vi "Set Data.vi"(8 "error in (no error)":errorcluster, 9 "Set Value":string, 10 "LogicName":string, 11 "PLC_Module in":refnum<class "PLC_Module.lvclass">) -> (0 "error out":errorcluster, 3 "PLC_Module out":refnum<class "PLC_Module.lvclass">)   [LabVIEW 2025, in "PLC_Module.lvlib" / "PLC_Module.lvclass"]
uses:
  PLC_Module.lvclass
  PLC_Module.lvclass/PLC_Module.ctl
  <vilib>/Utility/miscctls.llb/LVMapReplaceAction.ctl
  PLC_Abstr/PLC_Abstr Messages/Write Data Msg/Write Data Msg.lvclass/Write Data Msg.ctl
  <vilib>/ActorFramework/Message Enqueuer/Message Enqueuer.lvclass/Message Enqueuer.ctl
  b9a00cdf-f003-4314-8ef1-cc05cebe1eef.vi
  6056e4c1-ed78-404a-9ef6-920044df1d88.vi
  96e6804c-cbe1-4d7e-8e4f-31ab62afd4e7.vi
  108bd21b-5831-41ec-9599-3e5880a8ed08.vi
  effe1758-f8e4-496e-af8d-4484fbab5602.vi
  549d32eb-c80e-4b94-81c6-920abf9741ef.vi
  Write Configuration.vi
  Read Configuration.vi
  Read Connect.vi
  <vilib>/ActorFramework/Message Enqueuer/Enqueue.vi
  PLC_Abstr/PLC_Abstr Messages/Write Data Msg/Write Data Msg.lvclass
  <vilib>/JDP Science/JSONtext/JSON text to Variant.vi
  <vilib>/ActorFramework/Message Priority Queue/Priority Enqueue.vi
  <vilib>/JDP Science/JSONtext/LVClass Serializer/JSONtext LVClass Serializer.lvclass
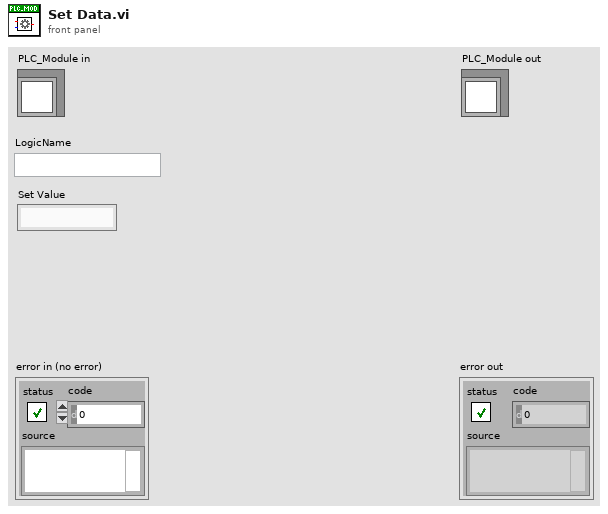
[diagram p1: front panel]
types:
  T1 = typedef "LVMapReplaceAction.ctl" = enum32{"Modify Entry only if found", "Add or Modify Entry", "Delete Entry"}
  T2 = typedef "PLC_Module.lvlib/PLC_Module.lvclass/PLC_Data_Config.ctl" = map{string, cluster{"Config":T3, "Get Value":string, "Set Value":string}}
  T3 = typedef "PLC_Module.lvlib/PLC_Module.lvclass/PLC_Data.ctl" = cluster{"Address":string, "Direction":enum16{"PC->PLC", "PLC->PC"}, "DataType":T4, "Description":string}
  T4 = typedef "PLC_Module.lvlib/PLC_Module.lvclass/PLC_Data_Type.ctl" = enum16{"Boolean", "Single Float", "U8", "U32", "U32_Array", "String"}
  T5 = cluster{"Config":T3, "Get Value":string, "Set Value":string}
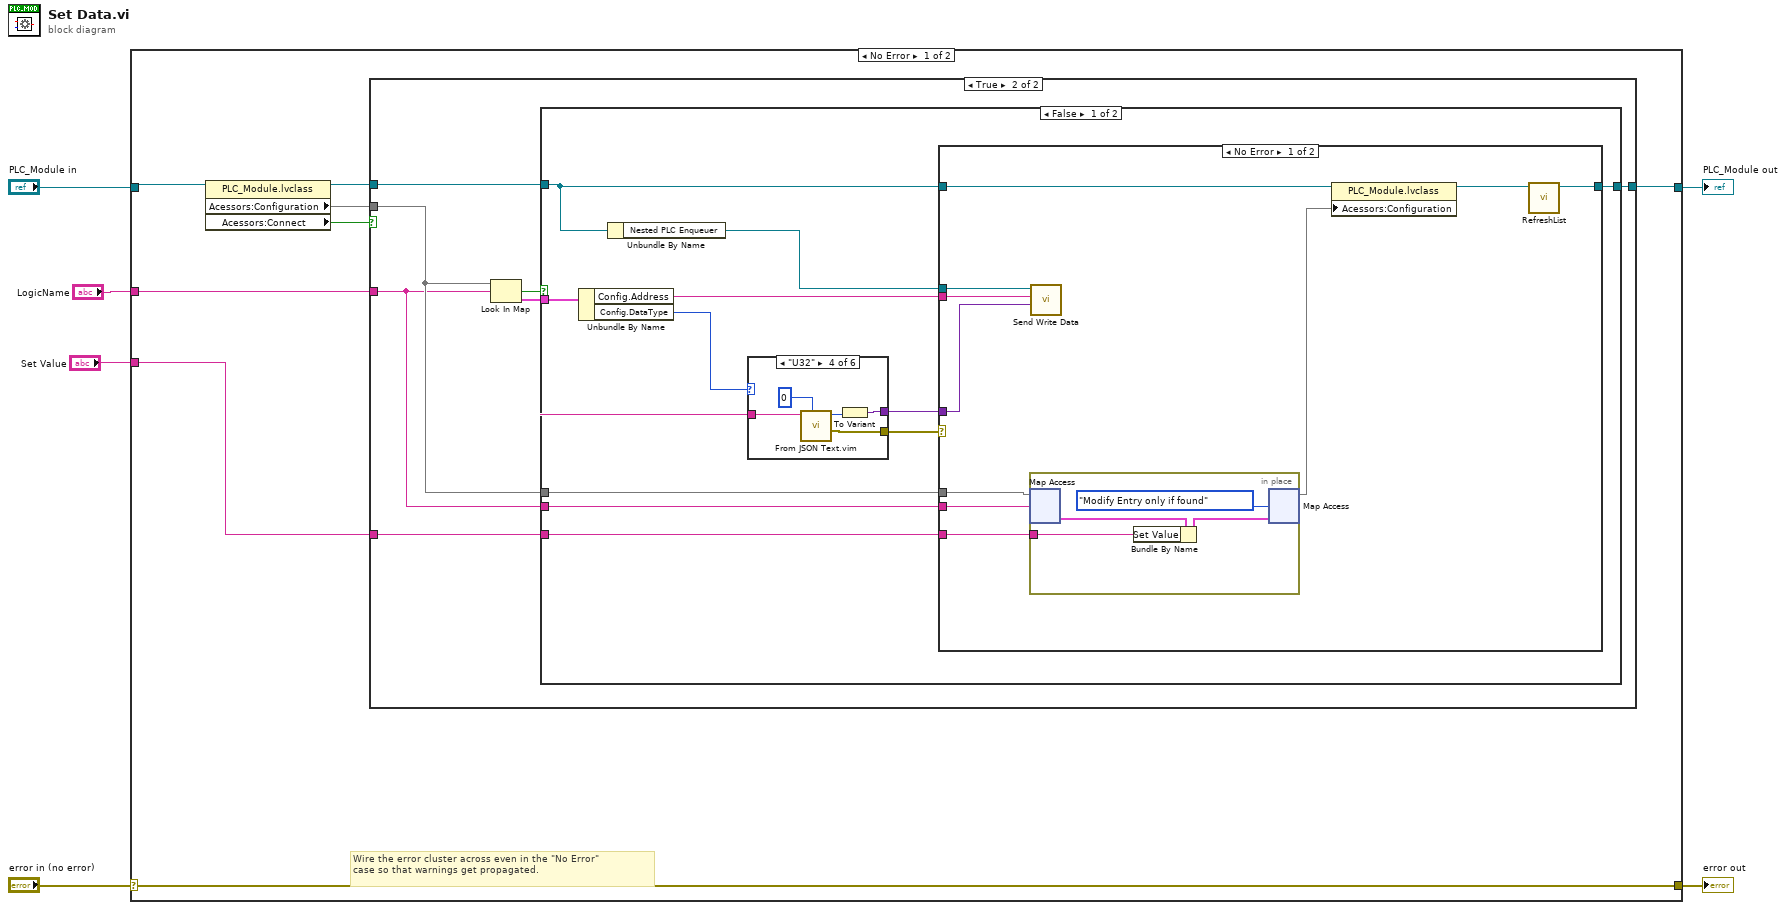
[diagram p0: block diagram]
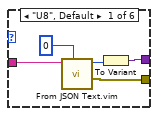
[diagram p4: hidden frame]
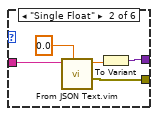
[diagram p5: hidden frame]
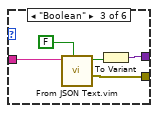
[diagram p6: hidden frame]
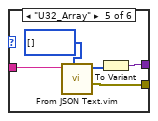
[diagram p7: hidden frame]
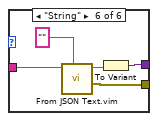
[diagram p8: hidden frame]
diagram:
  n1 = case shown="No Error" "error in (no error)" {
    selector: "error in (no error)" -> [w14 w81]
    tunnel: [w14 w81] -> w5
    tunnel: [w10 w80] -> w3
    tunnel: "PLC_Module in" -> [w13 w80]
    tunnel: "LogicName" -> [w9 _]
    tunnel: "Set Value" -> [w8 _]
    frame No Error {
      # "Wire the error cluster across even in the \"No Error\"\ncase so that warnings get propagated."
      n2 = property class="PLC_Module.lvclass"(reference=w13) -> (reference out=w12:refnum<class "PLC_Module.lvclass">, "Acessors:Configuration"=w11:T2, "Acessors:Connect"=w7:bool)  [unwired: 1 in, 1 out]
      n3 = case shown="True" w7 {
        tunnel: w12 -> [w15 w21]
        tunnel: w11 -> [_ w20]
        tunnel: [w15 w19] -> w10
        tunnel: w9 -> [_ w18]
        tunnel: w8 -> [_ w17]
        frame False {
        }
        frame True {
          n4 = Look In Map(map=w20, key=w18) -> (key not found?=w16:bool, value=w22:T5)  [unwired: 1 in]
          n5 = case shown="False" w16 {
            tunnel: w22 -> [w32 _]
            tunnel: w21 -> [w27 w79]
            tunnel: w20 -> [w26 _]
            tunnel: [w25 w79] -> w19
            tunnel: w18 -> [w24 _]
            tunnel: w17 -> [w23 _]
            frame False {
              n6 = Unbundle By Name(w32) -> ("Config.Address"=w31:string, "Config.DataType"=w30:T4)
              n7 = Unbundle By Name(w27) -> ("Nested PLC Enqueuer"=w33:refnum<class "Message Enqueuer.lvclass">)
              n8 = case shown="\"U32\"" w30 {
                tunnel: [w52 w57 w62 w67 w72 w77] -> w29
                tunnel: w23 -> [w53 w58 w63 w68 w73 w78]
                tunnel: [w49 w54 w59 w64 w70 w75] -> w28
                frame "U8", Default {
                  n9 = call "From JSON Text.vim"("Data Type and Default Value"=u8 0, "JSON"=w53) -> ("error out"=w52:errorcluster, "Data out"=w50:u8)  [unwired: 8 in]
                  n10 = To Variant(anything=w50) -> (Variant=w49:variant)
                }
                frame "Single Float" {
                  n11 = call "From JSON Text.vim"("Data Type and Default Value"=sgl 0.0, "JSON"=w58) -> ("error out"=w57:errorcluster, "Data out"=w55:sgl)  [unwired: 8 in]
                  n12 = To Variant(anything=w55) -> (Variant=w54:variant)
                }
                frame "Boolean" {
                  n13 = call "From JSON Text.vim"("Data Type and Default Value"=FALSE, "JSON"=w63) -> ("error out"=w62:errorcluster, "Data out"=w60:bool)  [unwired: 8 in]
                  n14 = To Variant(anything=w60) -> (Variant=w59:variant)
                }
                frame "U32" {
                  n15 = call "From JSON Text.vim"("Data Type and Default Value"=u32 0, "JSON"=w68) -> ("error out"=w67:errorcluster, "Data out"=w65:u32)  [unwired: 8 in]
                  n16 = To Variant(anything=w65) -> (Variant=w64:variant)
                }
                frame "U32_Array" {
                  n17 = call "From JSON Text.vim"("Data Type and Default Value"=u32[] [], "JSON"=w73) -> ("error out"=w72:errorcluster, "Data out"=w71:u32[])  [unwired: 8 in]
                  n18 = To Variant(anything=w71) -> (Variant=w70:variant)
                }
                frame "String" {
                  n19 = call "From JSON Text.vim"("Data Type and Default Value"="", "JSON"=w78) -> ("error out"=w77:errorcluster, "Data out"=w76:string)  [unwired: 8 in]
                  n20 = To Variant(anything=w76) -> (Variant=w75:variant)
                }
              }
              n21 = case shown="No Error" w29 {
                tunnel: w33 -> [w43 _]
                tunnel: w31 -> [w42 _]
                tunnel: w28 -> [w41 _]
                tunnel: w27 -> [w40 w48]
                tunnel: w26 -> [w39 _]
                tunnel: [w34 w48] -> w25
                tunnel: w24 -> [w38 _]
                tunnel: w23 -> [w37 _]
                frame No Error {
                  n22 = in-place {
                    in-place-border: w37 -> [w44]
                    n23 = in-place-map #1(w39, w38) -> (w47:T5)  [unwired: 1 in, 1 out]
                    n24 = Bundle By Name(cluster=w47, "Set Value"=w44) -> (w45:T5)
                    n25 = in-place-map #1(w45, LVMapReplaceAction."Modify Entry only if found" ("action")) -> (w36:T2)  [unwired: 2 out]
                  }
                  n26 = call "Send Write Data.vi"("Data"=w41, "Address"=w42, "Message Enqueuer"=w43) -> ()  [unwired: 7 in, 2 out]
                  n27 = property class="PLC_Module.lvclass"(reference=w40, "Acessors:Configuration"=w36) -> (reference out=w35:refnum<class "PLC_Module.lvclass">)  [unwired: 1 in, 1 out]
                  n28 = call "RefreshList.vi"("PLC_Module in"=w35) -> ("PLC_Module out"=w34:refnum<class "PLC_Module.lvclass">)  [unwired: 9 in, 1 out]
                }
                frame Error {
                }
              }
            }
            frame True {
            }
          }
        }
      }
    }
    frame Error {
    }
  }
  "error out" <- w5
  "PLC_Module out" <- w3
